vi "to string.vi"(8 "error in":errorcluster, 11 "J1939 configuration in":refnum<class "J1939 configuration.lvclass">) -> (0 "error out":errorcluster, 1 "data":string, 2 "version":string, 3 "J1939 configuration out":refnum<class "J1939 configuration.lvclass">)   [LabVIEW 2017, in "J1939 configuration.lvclass"]
doc: "Provides an interface for saving a module configuration to a file or other serialized data source. It is recommended that all children of this class store data in two sets--data required for its own initialization, and any data required for parent initialization--and that each implementation uses the <b>Call Parent Method</b> primitive to serialize parent information."
uses:
  J1939 configuration.lvclass
  J1939 configuration.lvclass/J1939 configuration.ctl
  current version.vi
  <vilib>/NI/Tag Bus Module Framework/module configuration/TBM module configuration.lvclass
  <vilib>/NI/Tag Bus Module Framework/channel/TBM channel.lvclass
  <vilib>/NI/Configuration Framework/serializable configuration/NISE_CEF_serializable configuration.lvclass
panel:
  out "concatenated string":string
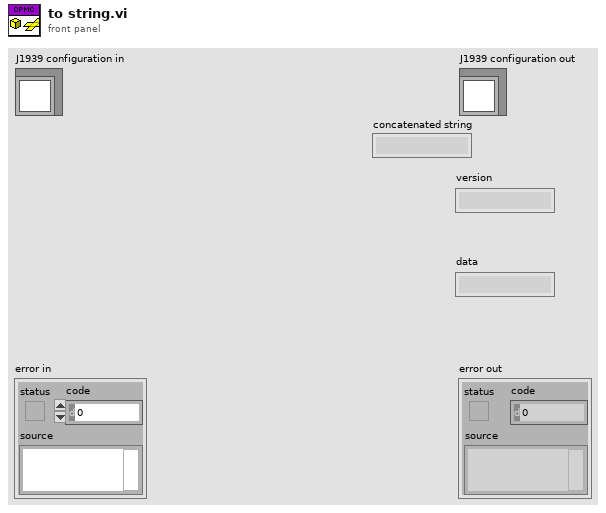
[diagram p1: front panel]
types:
  T1 = typedef "J1939 configuration.lvclass/Line.ctl" = cluster{"channel":refnum<class "TBM channel.lvclass">, "XNET Signal":refnum<k21>}
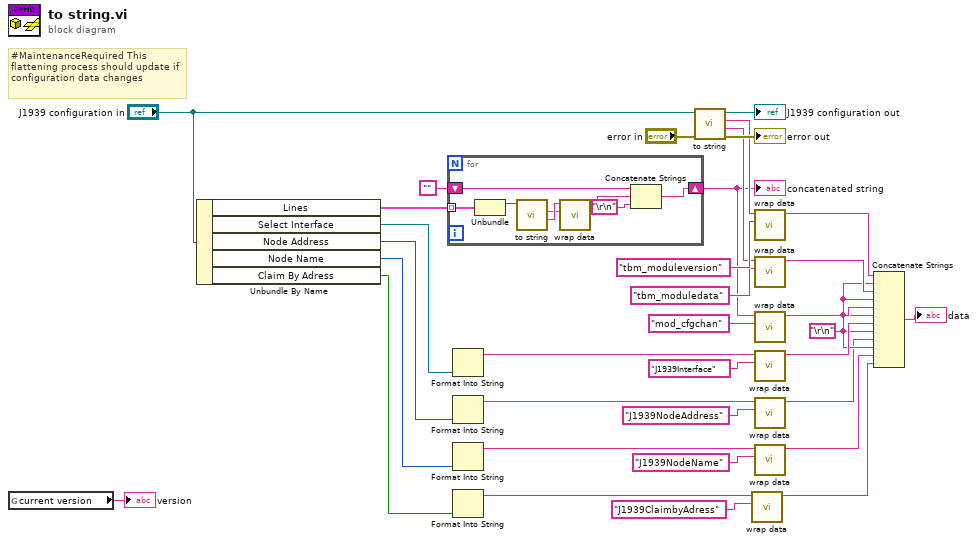
[diagram p0: block diagram]
diagram:
  w17 = "\r\n"
  # "#MaintenanceRequired This flattening process should update if configuration data changes"
  n1 = global read "current version.vi" "current version"() -> (→"version":string)
  n2 = Unbundle By Name("J1939 configuration in") -> ("Lines"=w21:T1[], "Select Interface"=w16:refnum<k21>, "Node Address"=w14:u8, "Node Name"=w11:u64, "Claim By Adress"=w1:bool)
  n3 = for {
    tunnel: w21 -> [w42] mode=indexing
    shift-right: [w35] -> w5
    shift-left: "" -> [w37]
    n4 = Unbundle(w42) -> ("channel"=w41:refnum<class "TBM channel.lvclass">)  [unwired: 1 out]
    n5 = call-dynamic "to string.vi"("channel in"=w41) -> ("channel data"=w40:string, "identifier"=w39:string)  [unwired: 7 in, 2 out]
    n6 = call <vilib>:"wrap data.vi"("identifier"=w39, "data to wrap"=w40) -> ("wrapped data"=w36:string)  [unwired: 9 in]
    n7 = Concatenate Strings(w37, w36, "\r\n") -> (w35:string)
  }
  "concatenated string" <- w5
  n8 = Format Into String(w16) -> (resulting string=w15:string)  [unwired: 3 in, 1 out]
  n9 = Format Into String(w14) -> (resulting string=w13:string)  [unwired: 3 in, 1 out]
  n10 = Format Into String(w11) -> (resulting string=w10:string)  [unwired: 3 in, 1 out]
  n11 = Format Into String(w1) -> (resulting string=w2:string)  [unwired: 3 in, 1 out]
  n12 = call-parent "to string.vi"("error in"="error in", "module configuration in"="J1939 configuration in") -> ("error out"=→"error out":errorcluster, "data"=w25:string, "version"=w26:string, "module configuration out"=→"J1939 configuration out":refnum<class "J1939 configuration.lvclass">)  [unwired: 6 in]
  n13 = call <vilib>:"wrap data.vi"("identifier"="J1939ClaimbyAdress", "data to wrap"=w2) -> ("wrapped data"=w3:string)  [unwired: 9 in]
  n14 = call <vilib>:"wrap data.vi"("identifier"="tbm_moduleversion" ("additional identifier"), "data to wrap"=w26) -> ("wrapped data"=w28:string)  [unwired: 9 in]
  n15 = call <vilib>:"wrap data.vi"("identifier"="tbm_moduledata" ("additional identifier"), "data to wrap"=w25) -> ("wrapped data"=w27:string)  [unwired: 9 in]
  n16 = call <vilib>:"wrap data.vi"("identifier"="mod_cfgchan", "data to wrap"=w5) -> ("wrapped data"=w22:string)  [unwired: 9 in]
  n17 = call <vilib>:"wrap data.vi"("identifier"="J1939Interface", "data to wrap"=w15) -> ("wrapped data"=w18:string)  [unwired: 9 in]
  n18 = call <vilib>:"wrap data.vi"("identifier"="J1939NodeAddress", "data to wrap"=w13) -> ("wrapped data"=w8:string)  [unwired: 9 in]
  n19 = call <vilib>:"wrap data.vi"("identifier"="J1939NodeName", "data to wrap"=w10) -> ("wrapped data"=w7:string)  [unwired: 9 in]
  n20 = Concatenate Strings(w28, w17, w27, w17, w22, w17, w18, w17, w8, w17, w7, w3) -> (→"data":string)
